vi "ParameterSet2CmdCluster.vi"(0 "CMDCluster In":T1, 7 "ParameterSet":string) -> (4 "CMDCluster Out":T1)   [LabVIEW 2013]
uses:
  TypeDef/Command Cluster.ctl
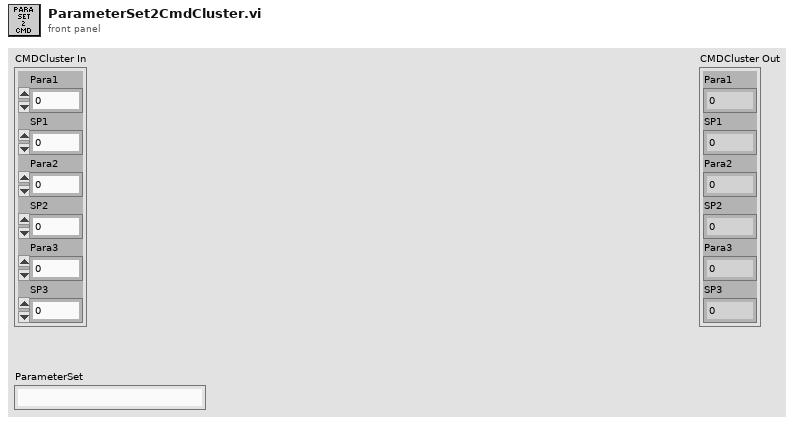
[diagram p1: front panel]
types:
  T1 = typedef "Command Cluster.ctl" = cluster{"Para1":i32, "SP1":dbl, "Para2":i32, "SP2":dbl, "Para3":i32, "SP3":dbl}
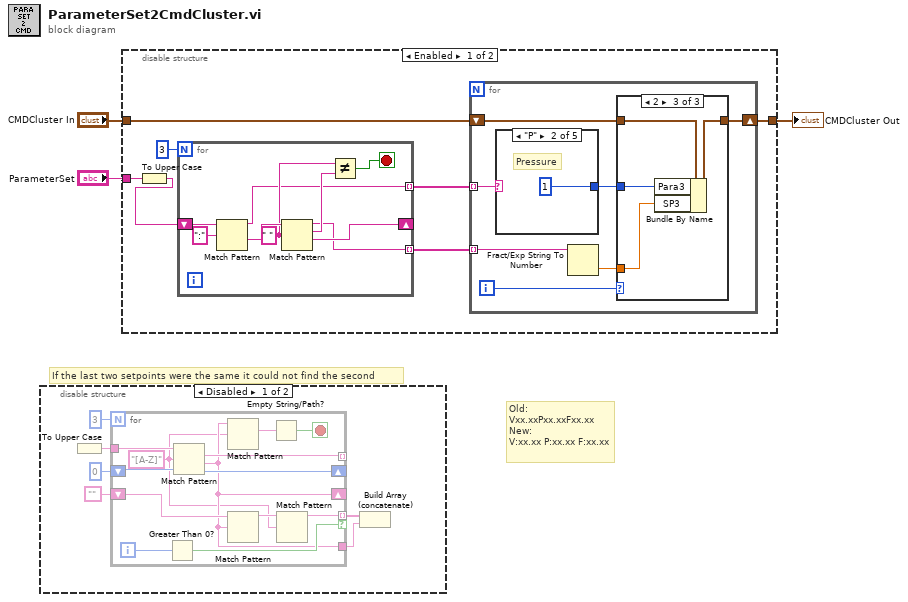
[diagram p0: block diagram]
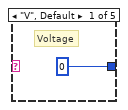
[diagram p2: hidden frame]
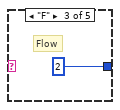
[diagram p3: hidden frame]
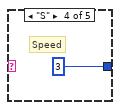
[diagram p4: hidden frame]
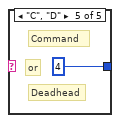
[diagram p5: hidden frame]
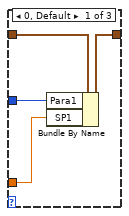
[diagram p6: hidden frame]
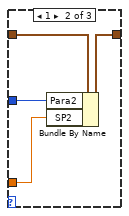
[diagram p7: hidden frame]
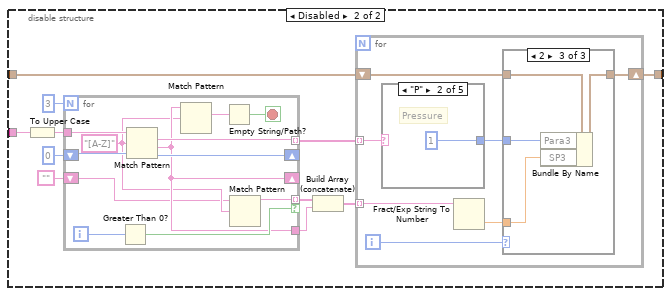
[diagram p8: hidden frame]
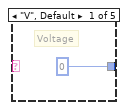
[diagram p9: hidden frame]
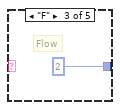
[diagram p10: hidden frame]
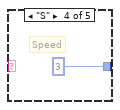
[diagram p11: hidden frame]
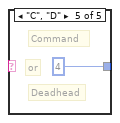
[diagram p12: hidden frame]
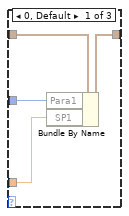
[diagram p13: hidden frame]
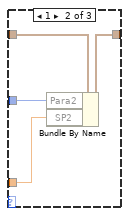
[diagram p14: hidden frame]
diagram:
  # "Old:\nVxx.xxPxx.xxFxx.xx\nNew:\nV:xx.xx P:xx.xx F:xx.xx"
  # "If the last two setpoints were the same it could not find the second"
  n1 = disable-structure shown="Disabled" {
    frame Disabled {
      n2 = To Upper Case() -> (0:w4:string)  [unwired: 1 in]
      n3 = for {
        N: 3 -> [_]
        tunnel: w4 -> [w23]
        shift-right: [w21] -> _
        shift-left: 0 ("offset past match") -> [w22]
        shift-right: [w14] -> _
        shift-left: "" -> [w20]
        tunnel: [w15] -> w7 mode=indexing if=w18
        tunnel: [w14] -> w8
        tunnel: [w17] -> w10 mode=indexing
        i -> [w19]
        stop <- w11 stop-if-true
        w13 = "[A-Z]" ("regular expression")
        n4 = Greater Than 0?(x=w19) -> (x > 0?=w18:bool)
        n5 = Match Pattern(string=w23, regular expression=w13, offset (0)=w22) -> (match substring=w17:string, after substring=w14:string, offset past match=w21:i32)  [unwired: 1 out]
        n6 = Match Pattern(string=w14, regular expression=w13) -> (match substring=w12:string)  [unwired: 1 in, 3 out]
        n7 = Match Pattern(string=w20, regular expression=w14) -> (before substring=w16:string)  [unwired: 1 in, 3 out]
        n8 = Empty String/Path?(string/path=w12) -> (empty?=w11:bool)
        n9 = Match Pattern(string=w16, regular expression=w13) -> (before substring=w15:string)  [unwired: 1 in, 3 out]
      }
      n10 = Build Array (concatenate)(w7, w8) -> ()  [unwired: 1 out]
    }
    frame Enabled {
    }
  }
  n11 = disable-structure shown="Enabled" {
    disable-tunnel: "ParameterSet" -> [w30 w74]
    disable-tunnel: "CMDCluster In" -> [w27 w65]
    disable-tunnel: [w26 w64] -> w1
    frame Enabled {
      n12 = To Upper Case(1:w30) -> (0:w25:string)
      n13 = for {
        N: 3 -> [_]
        shift-right: [w56] -> _
        shift-left: w25 -> [w63]
        tunnel: [w55] -> w24 mode=indexing
        tunnel: [w57] -> w28 mode=indexing
        stop <- w58 stop-if-true
        w60 = " " ("regular expression")
        n14 = Match Pattern(string=w63, regular expression=":") -> (before substring=w57:string, after substring=w61:string)  [unwired: 1 in, 2 out]
        n15 = Match Pattern(string=w61, regular expression=w60) -> (before substring=w55:string, match substring=w59:string, after substring=w56:string)  [unwired: 1 in, 1 out]
        n16 = Not Equal?(x=w60, y=w59) -> (x != y?=w58:bool)
      }
      n17 = for {
        tunnel: w24 -> [w36] mode=indexing
        tunnel: w28 -> [w34] mode=indexing
        shift-right: [w32] -> w26
        shift-left: w27 -> [w33]
        i -> [w37]
        n18 = case shown="\"P\"" w34 {
          tunnel: [0 ("Para1") 1 ("Para1") 2 ("Para1") 3 ("Para1") 4 ("Para1")] -> w31
          frame "V", Default {
            # "Voltage"
          }
          frame "P" {
            # "Pressure"
          }
          frame "F" {
            # "Flow"
          }
          frame "S" {
            # "Speed"
          }
          frame "C", "D" {
            # "or"
            # "Deadhead"
            # "Command"
          }
        }
        n19 = Fract/Exp String To Number(string=w36) -> (number=w35:dbl)  [unwired: 3 in, 1 out]
        n20 = case shown="2" w37 {
          tunnel: w35 -> [w43 w47 w51]
          tunnel: w33 -> [w46 w50 w54]
          tunnel: [w45 w49 w53] -> w32
          tunnel: w31 -> [w44 w48 w52]
          frame 0, Default {
            n21 = Bundle By Name(cluster=w46, "Para1"=w44, "SP1"=w43) -> (w45:T1)
          }
          frame 1 {
            n22 = Bundle By Name(cluster=w50, "Para2"=w48, "SP2"=w47) -> (w49:T1)
          }
          frame 2 {
            n23 = Bundle By Name(cluster=w54, "Para3"=w52, "SP3"=w51) -> (w53:T1)
          }
        }
      }
    }
    frame Disabled {
      n24 = To Upper Case(1:w74) -> (0:w73:string)
      n25 = for {
        N: 3 -> [_]
        tunnel: w73 -> [w110]
        shift-right: [w108] -> _
        shift-left: 0 ("offset past match") -> [w109]
        shift-right: [w103] -> _
        shift-left: "" -> [w99]
        tunnel: [w104] -> w70 mode=indexing if=w106
        tunnel: [w103] -> w69
        tunnel: [w105] -> w66 mode=indexing
        i -> [w107]
        stop <- w100 stop-if-true
        w102 = "[A-Z]" ("regular expression")
        n26 = Greater Than 0?(x=w107) -> (x > 0?=w106:bool)
        n27 = Match Pattern(string=w110, regular expression=w102, offset (0)=w109) -> (match substring=w105:string, after substring=w103:string, offset past match=w108:i32)  [unwired: 1 out]
        n28 = Match Pattern(string=w103, regular expression=w102) -> (match substring=w101:string)  [unwired: 1 in, 3 out]
        n29 = Empty String/Path?(string/path=w101) -> (empty?=w100:bool)
        n30 = Match Pattern(string=w99, regular expression=w102) -> (before substring=w104:string)  [unwired: 1 in, 3 out]
      }
      n31 = Build Array (concatenate)(w70, w69) -> (w67:string[])
      n32 = for {
        tunnel: w67 -> [w80] mode=indexing
        tunnel: w66 -> [w78] mode=indexing
        shift-right: [w76] -> w64
        shift-left: w65 -> [w77]
        i -> [w81]
        n33 = case shown="\"P\"" w78 {
          tunnel: [0 ("Para1") 1 ("Para1") 2 ("Para1") 3 ("Para1") 4 ("Para1")] -> w75
          frame "V", Default {
            # "Voltage"
          }
          frame "P" {
            # "Pressure"
          }
          frame "F" {
            # "Flow"
          }
          frame "S" {
            # "Speed"
          }
          frame "C", "D" {
            # "or"
            # "Deadhead"
            # "Command"
          }
        }
        n34 = Fract/Exp String To Number(string=w80) -> (number=w79:dbl)  [unwired: 3 in, 1 out]
        n35 = case shown="2" w81 {
          tunnel: w79 -> [w87 w91 w95]
          tunnel: w77 -> [w90 w94 w98]
          tunnel: [w89 w93 w97] -> w76
          tunnel: w75 -> [w88 w92 w96]
          frame 0, Default {
            n36 = Bundle By Name(cluster=w90, "Para1"=w88, "SP1"=w87) -> (w89:T1)
          }
          frame 1 {
            n37 = Bundle By Name(cluster=w94, "Para2"=w92, "SP2"=w91) -> (w93:T1)
          }
          frame 2 {
            n38 = Bundle By Name(cluster=w98, "Para3"=w96, "SP3"=w95) -> (w97:T1)
          }
        }
      }
    }
  }
  "CMDCluster Out" <- w1
